vi "Trigger Visible Write.vi"(4 "error in (no error)":errorcluster, 5 "Value":bool, 6 "Container State":T4, 7 "Display State In":T1) -> (0 "error out":errorcluster, 3 "Display State Out":T1)   [LabVIEW 2020, in "PXISlotGP.xctl"]
uses:
  PXISlotGP.xctl
  <vilib>/_xctls/Container State.ctl
  State.ctl
  PXISlot XControl/Connector Type.ctl
  AOAIRefs.ctl
  <vilib>/_xctls/XControlSupport.lvlib
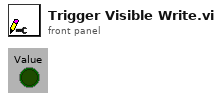
[diagram p1: front panel]
types:
  T1 = typedef "PXISlotGP.xctl/State.ctl" = cluster{"Connector Type":T2, "Hide unused":bool, "Trigger Visible":bool, "TabRef":refnum<vi>, "ConnRefs":refnum<vi>[], "PaneRef":refnum<vi>, "AOAIRefs":T3[], "TriggerRefs":refnum<vi>[], "check data":bool, "Name":string, "Events":cluster{"Type changed":refnum<user-event>}}
  T2 = typedef "Connector Type.ctl" = enum16{"None", "PXI-4461", "BNC-2110", "BNC-2090", "PXIe-4463", "PXIe-4464"}
  T3 = typedef "AOAIRefs.ctl" = cluster{"AORefs":refnum<vi>[], "AIRefs":refnum<vi>[]}
  T4 = typedef "XControlSupport.lvlib/Container State.ctl" = cluster{"Indicator?":bool, "Run Mode?":bool, " Refnum":refnum<vi>}
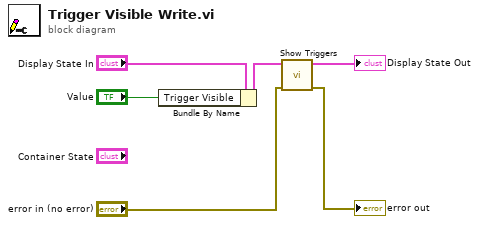
[diagram p0: block diagram]
diagram:
  n1 = Bundle By Name(cluster="Display State In", "Trigger Visible"="Value") -> (w3:T1)
  n2 = call "Show Triggers.vi"("error in (no error)"="error in (no error)", "Display State In"=w3) -> ("error out"=→"error out":errorcluster, "Display State Out"=→"Display State Out":T1)  [unwired: 8 in]
